vi "ke37xx Enable-Disable DAC Outputs.vi"(8 "error in (no error)":errorcluster, 9 "Enable/Disable Output (Disable)":bool, 10 "Channel":string, 11 "VISA Resource Name":refnum<visa-resource-name>) -> (0 "error out":errorcluster, 3 "VISA Resource Name Out":refnum<visa-resource-name>)   [LabVIEW 2009, in "Keithley 3700 Series.lvlib"]
doc: "This VI enables or disables the output for DAC channels."
uses:
  <instrlib>/Keithley 3706/Keithley 3700 Series.lvlib
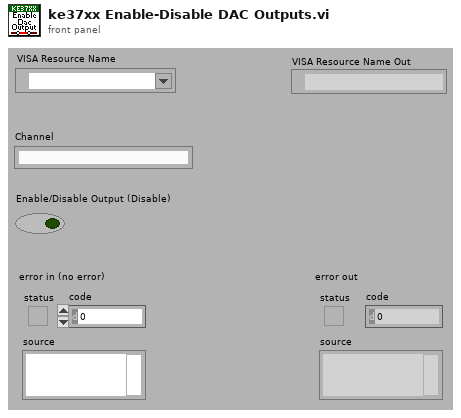
[diagram p1: front panel]
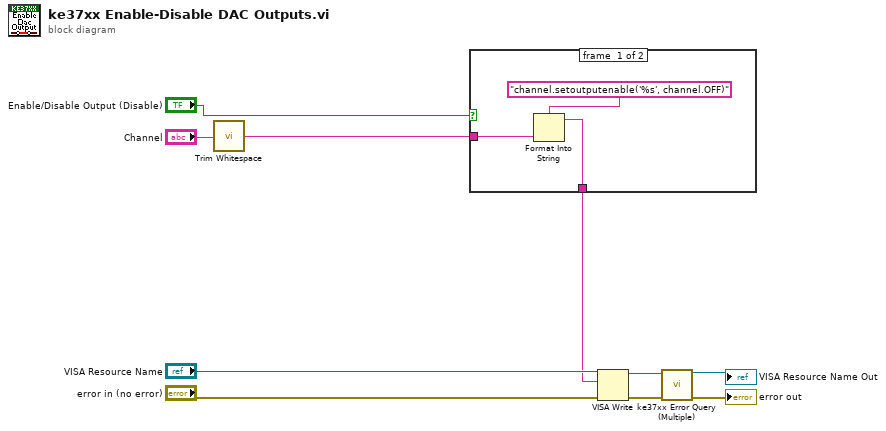
[diagram p0: block diagram]
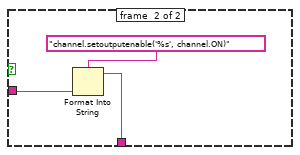
[diagram p2: hidden frame]
diagram:
  n1 = call <vilib>:"Trim Whitespace.vi"("string"="Channel") -> ("trimmed string"=w4:string)  [unwired: 1 in]
  n2 = case shown="False" "Enable/Disable Output (Disable)" {
    tunnel: [w12 w14] -> w6
    tunnel: w4 -> [w11 w15]
    frame #0 {
      n3 = Format Into String(format string="channel.setoutputenable('%s', channel.OFF)", w11) -> (resulting string=w12:string)  [unwired: 2 in, 1 out]
    }
    frame #1 {
      n4 = Format Into String(format string="channel.setoutputenable('%s', channel.ON)", w15) -> (resulting string=w14:string)  [unwired: 2 in, 1 out]
    }
  }
  n5 = VISA Write(VISA resource name="VISA Resource Name", write buffer=w6, error in (no error)="error in (no error)") -> (VISA resource name out=w3:refnum<visa-resource-name>, error out=w2:errorcluster)  [unwired: 1 out]
  n6 = call <instrlib>:"ke37xx Error Query (Multiple).vi"("VISA resource name"=w3, "error in (no error)"=w2) -> ("VISA resource name out"=→"VISA Resource Name Out":refnum<visa-resource-name>, "error out"=→"error out":errorcluster)  [unwired: 12 out]
